vi "Async.Processes.Report.vi"(8 "Error":errorcluster, 10 "Stop on Error?":bool, 11 "Process in":refnum<class "Process.lvclass">) -> (2 "Stop":bool, 3 "Process out":refnum<class "Process.lvclass">)   [LabVIEW 2015, in "VS Inline Async API.lvlib" / "Process.lvclass"]
uses:
  Process.lvclass
  Process.lvclass/Process.ctl
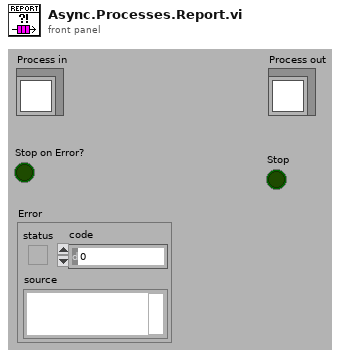
[diagram p1: front panel]
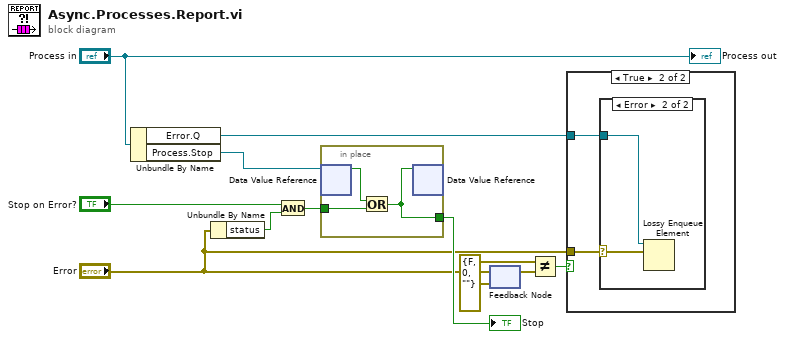
[diagram p0: block diagram]
diagram:
  n1 = Unbundle By Name("Process in") -> ("Error.Q"=w8:refnum<queue>, "Process.Stop"=w2:refnum<data-value>)
  n2 = Unbundle By Name("Error") -> ("status"=w6:bool)
  n3 = And(x="Stop on Error?", y=w6) -> (x .and. y?=w5:bool)
  n4 = in-place {
    in-place-border: [w12] -> w4
    in-place-border: w5 -> [w13]
    n5 = in-place-dvr #1(w2) -> (w14:bool)  [unwired: 1 out]
    n6 = Or(x=w14, y=w13) -> (x .or. y?=w12:bool)
    n7 = in-place-dvr #1(w12) -> ()  [unwired: 2 out]
  }
  "Stop" <- w4
  n8 = feedback #2(errorcluster {"status"=FALSE, "code"=0, "source"=""} ("Error")) -> (w10:errorcluster)
  n9 = feedback-in #2("Error") -> ()
  n10 = Not Equal?(x="Error", y=w10) -> (x != y?=w11:bool)
  n11 = case shown="True" w11 {
    tunnel: w8 -> [_ w16]
    tunnel: "Error" -> [_ w15]
    frame False {
    }
    frame True {
      n12 = case shown="Error" w15 {
        selector: w15 -> [_ w17]
        tunnel: w16 -> [_ w18]
        frame No Error {
        }
        frame Error {
          n13 = Lossy Enqueue Element(queue=w18, element=w17) -> ()  [unwired: 1 in, 4 out]
        }
      }
    }
  }
  "Process out" <- "Process in"
